vi "Check if Error Occurred.vi"(8 "error in (no error)":errorcluster, 11 "Response header":string) -> (0 "error out":errorcluster, 2 "500 Error":bool, 3 "Error Occurred":bool)   [LabVIEW 2015, in "NI_AWS_Core.lvlib" / "HTTP Request.lvclass"]
doc: "Check the response header to see if there was an error.\nIf an error is found, the AWS_S3_Get_Call_Result.vi may get the details from the response body."
uses:
  HTTP Request.lvclass
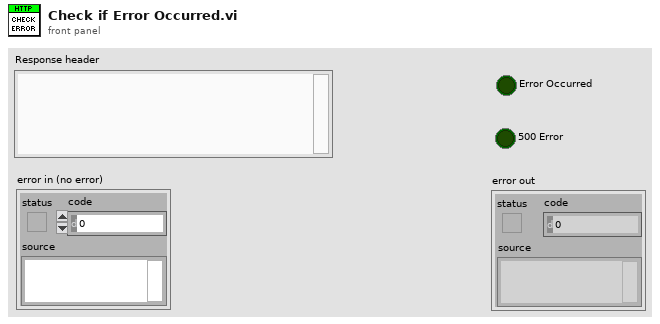
[diagram p1: front panel]
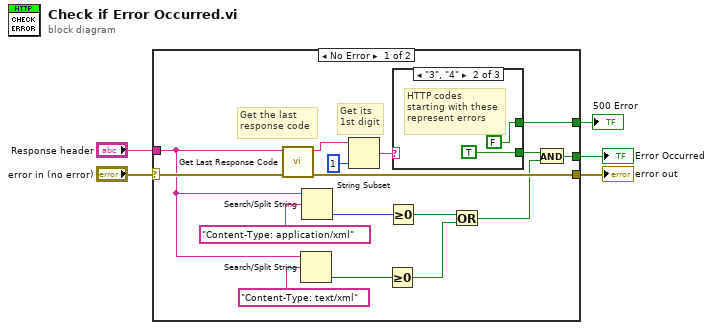
[diagram p0: block diagram]
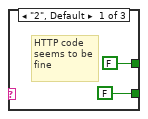
[diagram p2: hidden frame]
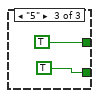
[diagram p3: hidden frame]
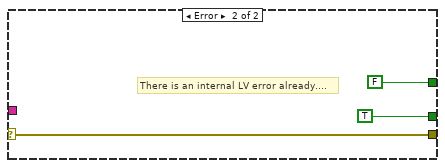
[diagram p4: hidden frame]
diagram:
  n1 = case shown="No Error" "error in (no error)" {
    selector: "error in (no error)" -> [w17 w30]
    tunnel: [w16 w30] -> w3
    tunnel: "Response header" -> [w9 _]
    tunnel: [w18 TRUE] -> w2
    tunnel: [w11 FALSE] -> w1
    frame No Error {
      # "Get its\n1st digit"
      # "Get the last\nresponse code"
      n2 = call "Get Last Response Code.vi"("error in (no error)"=w17, "Response header"=w9) -> ("error out"=w16:errorcluster, "Response code (last)"=w15:string)  [unwired: 8 in]
      n3 = Search/Split String(string=w9, search string/char (-)="Content-Type: text/xml") -> (offset of match=w10:i32)  [unwired: 1 in, 2 out]
      n4 = Search/Split String(string=w9, search string/char (-)="Content-Type: application/xml") -> (offset of match=w20:i32)  [unwired: 1 in, 2 out]
      n5 = String Subset(string=w15, length (rest)=1 ("length (rest)")) -> (substring=w14:string)  [unwired: 1 in]
      n6 = Greater Or Equal To 0?(x=w10) -> (x >= 0?=w6:bool)
      n7 = Greater Or Equal To 0?(x=w20) -> (x >= 0?=w12:bool)
      n8 = case shown="\"3\", \"4\"" w14 {
        tunnel: [FALSE TRUE TRUE] -> w19
        tunnel: [FALSE FALSE TRUE] -> w11
        frame "2", Default {
          # "HTTP code\nseems to be\nfine"
        }
        frame "3", "4" {
          # "HTTP codes\nstarting with these\nrepresent errors"
        }
        frame "5" {
        }
      }
      n9 = Or(x=w12, y=w6) -> (x .or. y?=w7:bool)
      n10 = And(x=w19, y=w7) -> (x .and. y?=w18:bool)
    }
    frame Error {
      # "There is an internal LV error already...."
    }
  }
  "Error Occurred" <- w2
  "error out" <- w3
  "500 Error" <- w1
